vi "Stop Core.vi"(10 "final error code":i32, 11 "Transfer Beginner in":refnum<class "Transfer Beginner.lvclass">) -> (3 "Transfer Beginner out":refnum<class "Transfer Beginner.lvclass">)   [LabVIEW 2020, in "CANopen.lvlib" / "SDO Manager.lvlib" / "Transfer Beginner.lvlib" / "Transfer Beginner.lvclass"]
doc: "<p>(<strong>Filename</strong>: <span class=\"dnl\">Actor Framework.lvlib:Actor.lvclass:Stop Core.vi</span>)</p>\n<p>Defines what the actor does before it stops. Use the <strong>final error code</strong> input to determine whether the actor shut down in response to an error.</p>\n<p>By default, this method passes the Stop message along to all <a href=\"nihelplauncher://docs/csh?context=lvcore_lvcomm_af_launch_nested_actor\">auto-stop nested actors</a>. A descendant class may override this method to define additional behavior, such as shutting down any processes the actor initiated in its override of the <a href=\"nihelplauncher://docs/csh?context=lvcore_lvcomm_af_actor_core\">Actor Core</a> method.</p>"
uses:
  Transfer Beginner.lvclass
  Transfer Beginner.lvclass/Transfer Beginner.ctl
  <vilib>/ActorFramework/Actor/Actor.lvclass
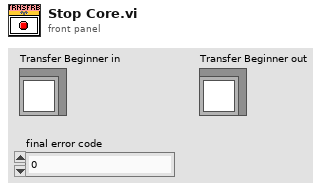
[diagram p1: front panel]
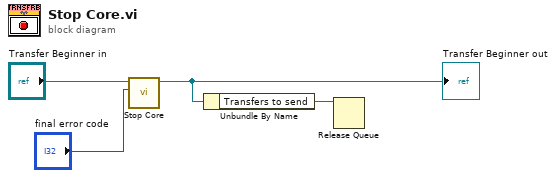
[diagram p0: block diagram]
diagram:
  n1 = call-parent "Stop Core.vi"("final error code"="final error code", "Actor in"="Transfer Beginner in") -> ("Actor out"=w2:refnum<class "Transfer Beginner.lvclass">)  [unwired: 9 in]
  "Transfer Beginner out" <- w2
  n2 = Unbundle By Name(w2) -> ("Transfers to send"=w1:refnum<queue>)
  n3 = Release Queue(queue=w1) -> ()  [unwired: 2 in, 3 out]
